vi "Update Front Panel.vi"(7 "Main References":T2, 8 "error in (no error)":errorcluster, 10 "input cluster":T1) -> (0 "error out":errorcluster)   [LabVIEW 2010]
uses:
  Main Refs.ctl
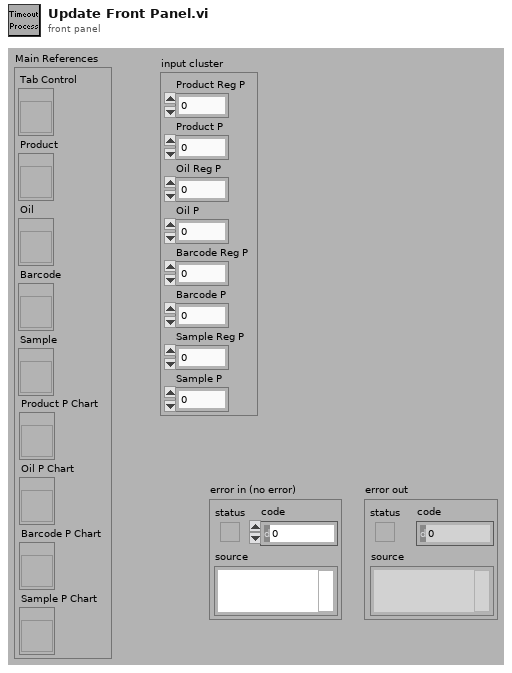
[diagram p1: front panel]
types:
  T1 = cluster{"Product Reg P":dbl, "Product P":dbl, "Oil Reg P":dbl, "Oil P":dbl, "Barcode Reg P":dbl, "Barcode P":dbl, "Sample Reg P":dbl, "Sample P":dbl}
  T2 = typedef "Main Refs.ctl" = cluster{"Tab Control":refnum<vi>, "Product":refnum<vi>, "Oil":refnum<vi>, "Barcode":refnum<vi>, "Sample":refnum<vi>, "Product P Chart":refnum<vi>, "Oil P Chart":refnum<vi>, "Barcode P Chart":refnum<vi>, "Sample P Chart":refnum<vi>}
  T3 = cluster{"Pump":bool, "Regulator":dbl, "Pressure Sensor":dbl, "Regulator Pressure Sensor":dbl, "Valve Control":bool[]}
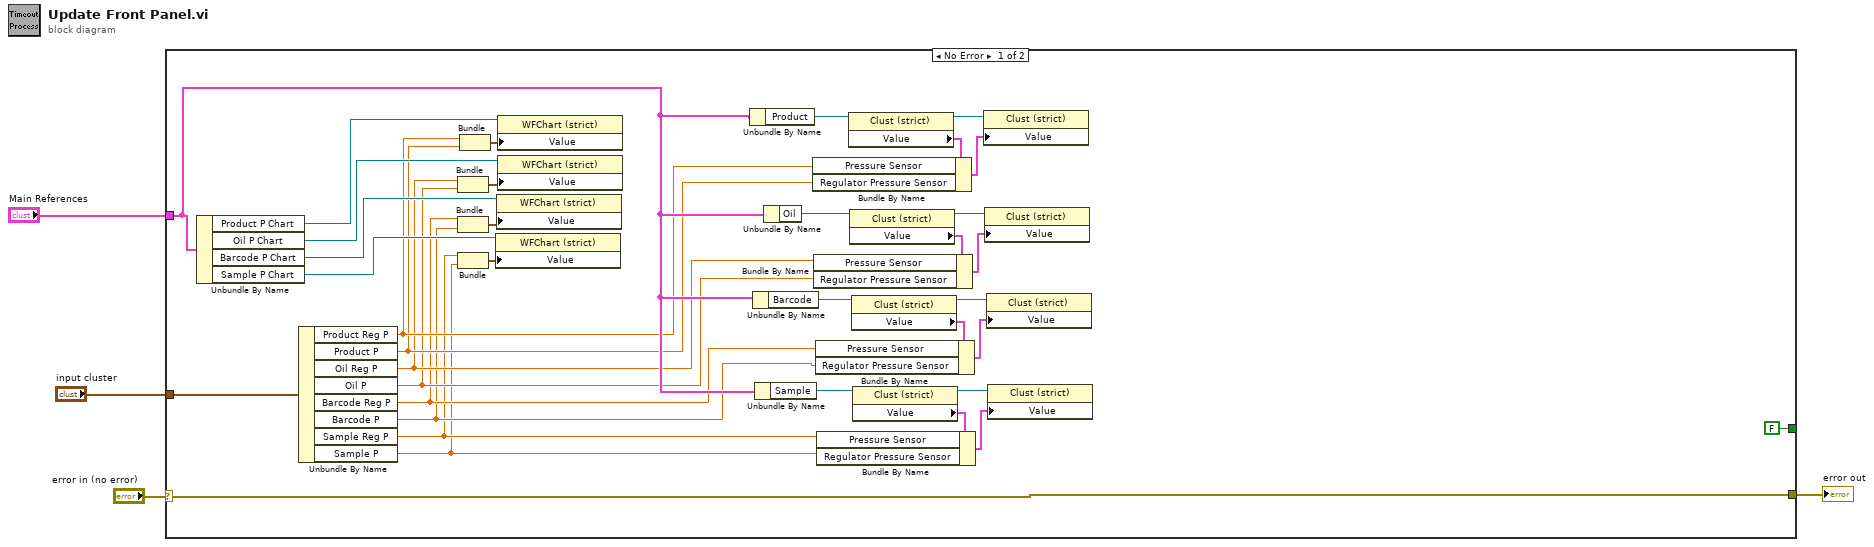
[diagram p0: block diagram]
diagram:
  n1 = case shown="No Error" "error in (no error)" {
    selector: "error in (no error)" -> [w6 w41]
    tunnel: [w6 w41] -> w3
    tunnel: [FALSE ("data") _] -> _
    tunnel: "Main References" -> [w19 _]
    tunnel: "input cluster" -> [w5 _]
    frame No Error {
      n2 = Unbundle By Name(w19) -> ("Product P Chart"=w38:refnum<vi>, "Oil P Chart"=w34:refnum<vi>, "Barcode P Chart"=w33:refnum<vi>, "Sample P Chart"=w32:refnum<vi>)
      n3 = Unbundle By Name(w5) -> ("Product Reg P"=w18:dbl, "Product P"=w17:dbl, "Oil Reg P"=w16:dbl, "Oil P"=w15:dbl, "Barcode Reg P"=w14:dbl, "Barcode P"=w13:dbl, "Sample Reg P"=w12:dbl, "Sample P"=w11:dbl)
      n4 = Bundle("Oil Reg P"=w16, "Oil P"=w15) -> (w37:cluster{"Oil Reg P":dbl, "Oil P":dbl})  [unwired: 1 in]
      n5 = Bundle("Barcode Reg P"=w14, "Barcode P"=w13) -> (w36:cluster{"Barcode Reg P":dbl, "Barcode P":dbl})  [unwired: 1 in]
      n6 = Bundle("Sample Reg P"=w12, "Sample P"=w11) -> (w35:cluster{"Sample Reg P":dbl, "Sample P":dbl})  [unwired: 1 in]
      n7 = Bundle("Product Reg P"=w18, "Product P"=w17) -> (w39:cluster{"Product Reg P":dbl, "Product P":dbl})  [unwired: 1 in]
      n8 = property class="WFChart (strict)"(reference=w32, "Value"=w35) -> ()  [unwired: 1 in, 2 out]
      n9 = property class="WFChart (strict)"(reference=w33, "Value"=w36) -> ()  [unwired: 1 in, 2 out]
      n10 = property class="WFChart (strict)"(reference=w38, "Value"=w39) -> ()  [unwired: 1 in, 2 out]
      n11 = property class="WFChart (strict)"(reference=w34, "Value"=w37) -> ()  [unwired: 1 in, 2 out]
      n12 = Unbundle By Name(w19) -> ("Product"=w25:refnum<vi>)
      n13 = Unbundle By Name(w19) -> ("Barcode"=w26:refnum<vi>)
      n14 = Unbundle By Name(w19) -> ("Sample"=w20:refnum<vi>)
      n15 = Unbundle By Name(w19) -> ("Oil"=w31:refnum<vi>)
      n16 = property class="Clust (strict)"(reference=w25) -> (reference out=w10:refnum<vi>, "Value"=w24:T3)  [unwired: 1 in, 1 out]
      n17 = Bundle By Name(cluster=w24, "Pressure Sensor"=w18, "Regulator Pressure Sensor"=w17) -> (w23:T3)
      n18 = property class="Clust (strict)"(reference=w31) -> (reference out=w9:refnum<vi>, "Value"=w30:T3)  [unwired: 1 in, 1 out]
      n19 = Bundle By Name(cluster=w30, "Pressure Sensor"=w16, "Regulator Pressure Sensor"=w15) -> (w29:T3)
      n20 = property class="Clust (strict)"(reference=w26) -> (reference out=w8:refnum<vi>, "Value"=w27:T3)  [unwired: 1 in, 1 out]
      n21 = Bundle By Name(cluster=w27, "Pressure Sensor"=w14, "Regulator Pressure Sensor"=w13) -> (w28:T3)
      n22 = property class="Clust (strict)"(reference=w20) -> (reference out=w7:refnum<vi>, "Value"=w21:T3)  [unwired: 1 in, 1 out]
      n23 = Bundle By Name(cluster=w21, "Pressure Sensor"=w12, "Regulator Pressure Sensor"=w11) -> (w22:T3)
      n24 = property class="Clust (strict)"(reference=w10, "Value"=w23) -> ()  [unwired: 1 in, 2 out]
      n25 = property class="Clust (strict)"(reference=w9, "Value"=w29) -> ()  [unwired: 1 in, 2 out]
      n26 = property class="Clust (strict)"(reference=w8, "Value"=w28) -> ()  [unwired: 1 in, 2 out]
      n27 = property class="Clust (strict)"(reference=w7, "Value"=w22) -> ()  [unwired: 1 in, 2 out]
    }
    frame Error {
    }
  }
  "error out" <- w3
